vi "Table Stage GUI.vi"() -> ()   [LabVIEW 2014]
uses:
  Controls/Translation Stage Types.ctl
  Controls/Queue Manager Actions.ctl
  Controls/MessagePacket.ctl
  Controls/QueueNames.ctl
panel:
  in  "Control Panel":T1(tab)
  in  "Table Stage Motion Controls":enum32{"Table Stage Controls"}(tab)
  in  "X":dbl
  in  "Y":dbl
  in  "Z":dbl
  in  "dZ":dbl=0.1 min=0.1 step=0.1
  in  "dY":dbl=0.1 min=0.1 step=0.1
  in  "dX":dbl=0.1 min=0.1 step=0.1
  in  "+Y":bool
  in  "-X":bool
  in  "+X":bool
  in  "-Y":bool
  in  "+Z":bool
  in  "-Z":bool
  out "X Stage":bool
  out "Y Stage":bool
  out "Z Stage":bool
  in  "Mosaic Quick Nav.":bool[][](array[boolean])
  in  "X Stage 4":T2 caption="Device Type"
  in  "X Stage 3":T2 caption="Device Type"
  in  "Home 3":bool caption="Home"
  in  "Home 2":bool caption="Home"
  in  "Home":bool
  in  "Reconnect Z":bool caption="Reconnect"
  in  "Reconnect Y":bool caption="Reconnect"
  in  "Reconnect X":bool caption="Reconnect"
  in  "X Stage 2":T2 caption="Device Type"
  in  "Center Galvos":bool
  out "Error Out":errorcluster
  in  "Error In":errorcluster
  # "Stage Controls"
  # "XYZ Axis Control"
  # "Current Postion"
  # "X STAGE SETTINGS"
  # "Y STAGE SETTINGS"
  # "Z STAGE SETTINGS"
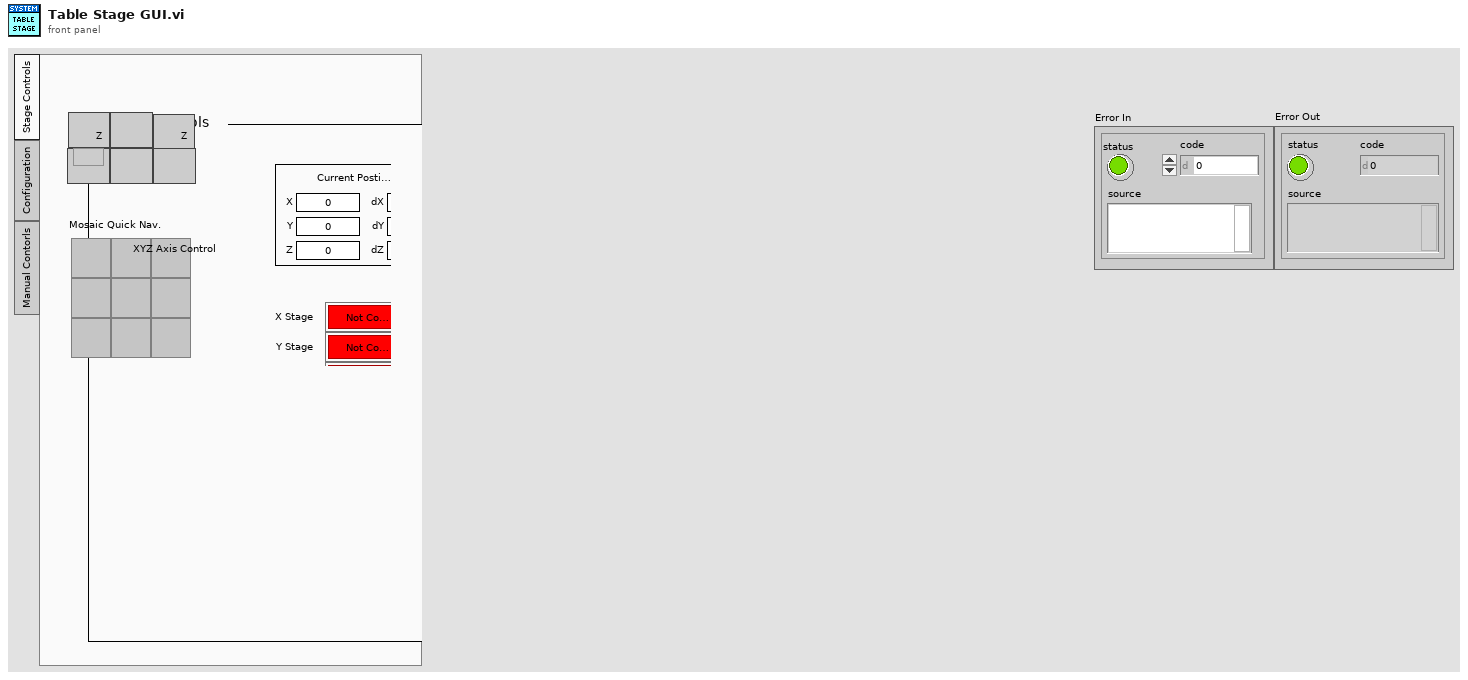
[diagram p1: front panel]
types:
  T1 = enum32{"Stage Controls", "Configuration", "Manual Contorls"}
  T2 = typedef "Translation Stage Types.ctl" = enum16{"None", "Thorlabs LTS", "Thorlabs MLJ"}
  T3 = typedef "MessagePacket.ctl" = cluster{"Message":string, "Parameter":variant}
  T4 = typedef "QueueNames.ctl" = enum16{"Main GUI", "Main Scan Processor", "Main Display", "Main Table Stage GUI", "Main Table Stage Proc."}
  T5 = typedef "Queue Manager Actions.ctl" = enum16{"Init", "Enqueue", "Enqueue All", "Preview Queue", "Dequeue", "Get Status", "Flush Queue", "Flush All Queues", "Release All Queues", "Release Queue"}
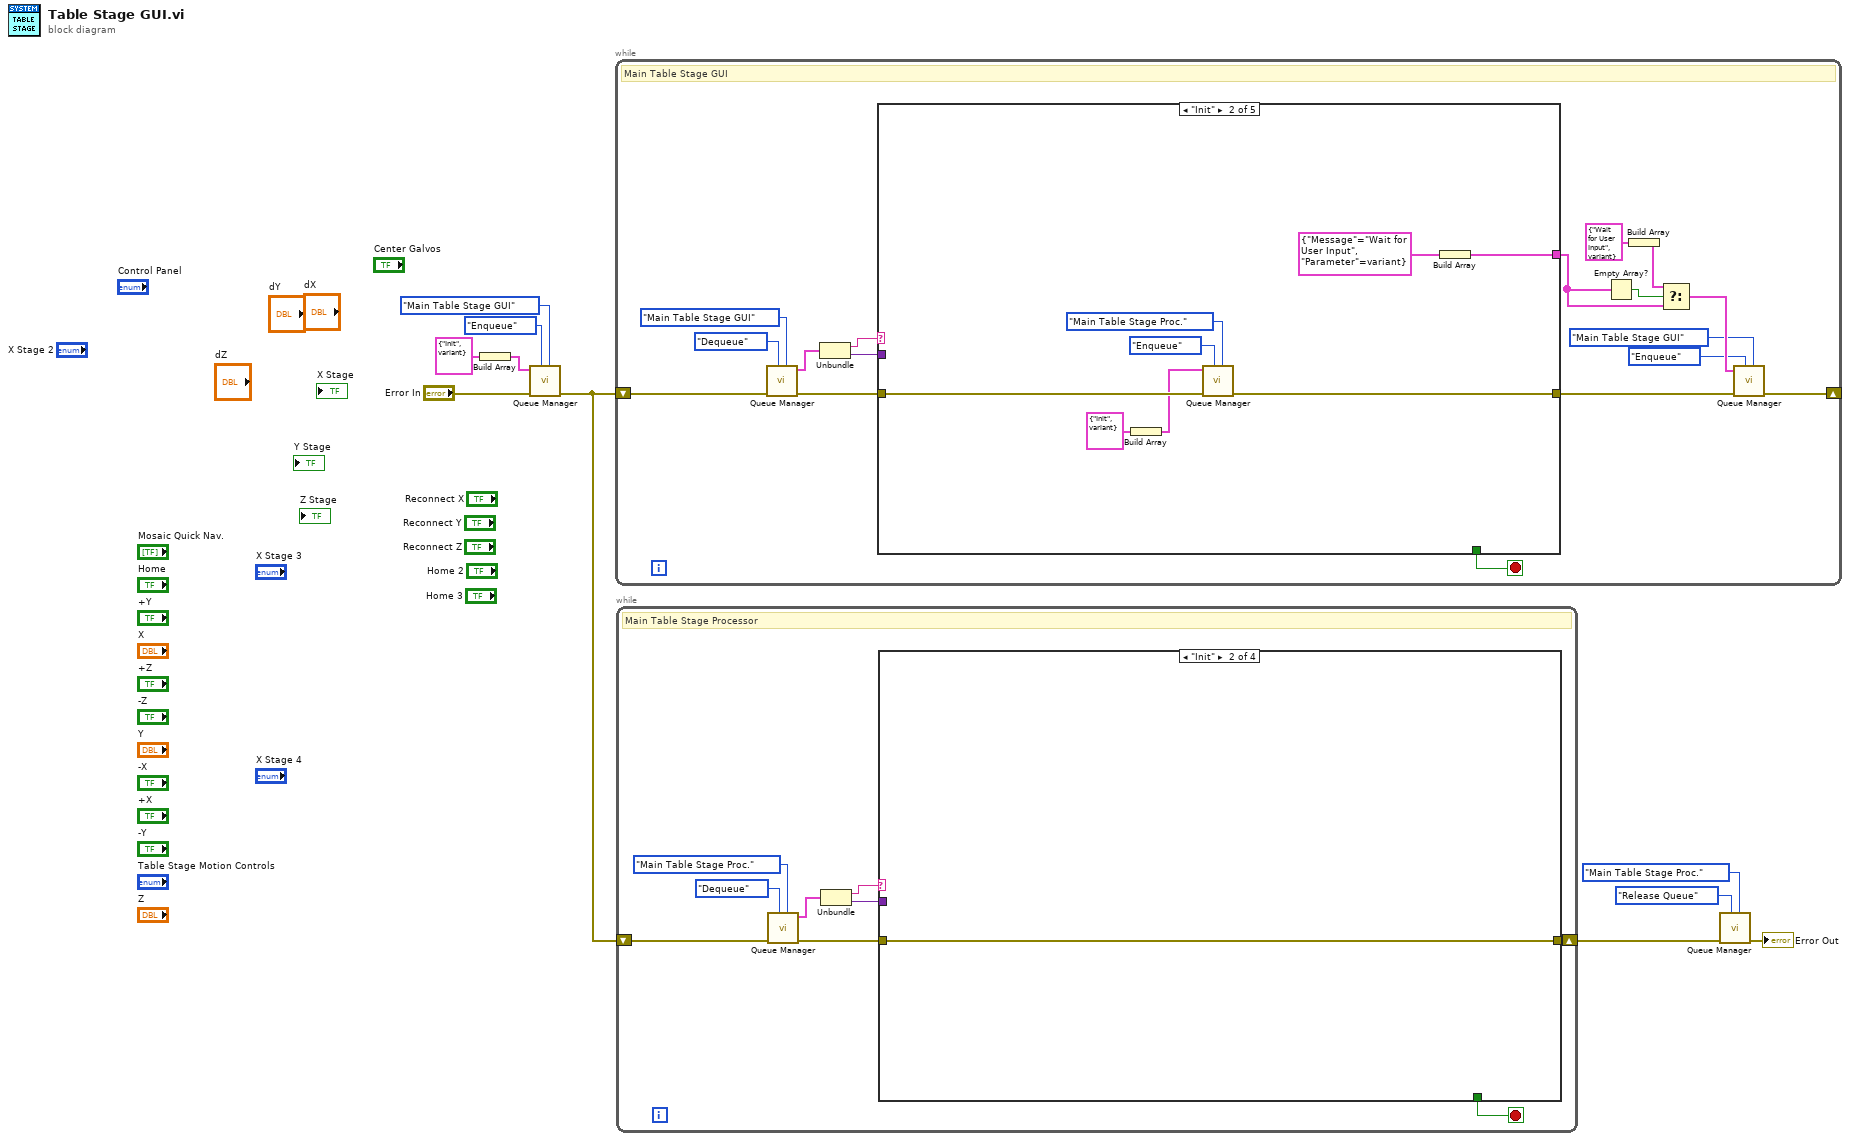
[diagram p0: block diagram]
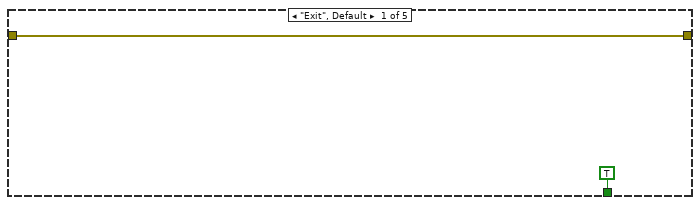
[diagram p2: hidden frame]
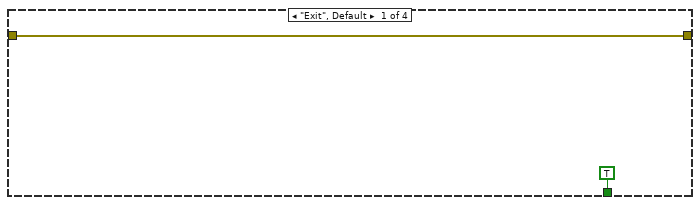
[diagram p6: hidden frame]
diagram:
  n1 = Build Array(T3 {"Message"="Init", "Parameter"=variant} ("Message Packet [In]")) -> (w1:T3[])
  n2 = call "Queue Manager.vi"("Queue Name"=QueueNames."Main Table Stage GUI", "Action"=Queue_Manager_Actions."Enqueue", "Error In"="Error In", "Message Packet Array"=w1) -> ("Error Out"=w3:errorcluster)  [unwired: 5 in, 2 out]
  n3 = while {
    shift-right: [w18] -> _
    shift-left: w3 -> [w25]
    stop <- w19 stop-if-true
    # "Main Table Stage GUI"
    n4 = call "Queue Manager.vi"("Queue Name"=QueueNames."Main Table Stage GUI", "Action"=Queue_Manager_Actions."Dequeue", "Error In"=w25) -> ("Error Out"=w24:errorcluster, "Message Packet [Out]"=w23:T3)  [unwired: 6 in, 1 out]
    n5 = Unbundle(w23) -> ("Message"=w22:string, "Parameter"=w21:variant)
    n6 = case shown="\"Init\"" w22 {
      tunnel: w24 -> [w28 w37 w38 w39 w40]
      tunnel: w21 -> [_ _ _ _ _]
      tunnel: [w28 w34 w38 w39 w40] -> w20
      tunnel: [TRUE _ _ _ _] -> w19
      tunnel: [_ w35 _ _ _] -> w11
      frame "Exit", Default {
      }
      frame "Init" {
        n7 = Build Array(T3 {"Message"="Init", "Parameter"=variant} ("Message Packet [In]")) -> (w30:T3[])
        n8 = call "Queue Manager.vi"("Queue Name"=QueueNames."Main Table Stage Proc.", "Action"=Queue_Manager_Actions."Enqueue", "Error In"=w37, "Message Packet Array"=w30) -> ("Error Out"=w34:errorcluster)  [unwired: 5 in, 2 out]
        n9 = Build Array(T3 {"Message"="Wait for User Input", "Parameter"=variant} ("Message Packet [In]")) -> (w35:T3[])
      }
      frame "Wait for User Input" {
      }
      frame "Init Hardware" {
      }
      frame "Idle" {
      }
    }
    n10 = Empty Array?(array=w11) -> (empty?=w17:bool)
    n11 = Build Array(T3 {"Message"="Wait for User Input", "Parameter"=variant} ("Message Packet [In]")) -> (w15:T3[])
    n12 = Select(t=w15, s=w17, f=w11) -> (s? t:f=w14:T3[])
    n13 = call "Queue Manager.vi"("Queue Name"=QueueNames."Main Table Stage GUI", "Action"=Queue_Manager_Actions."Enqueue", "Error In"=w20, "Message Packet Array"=w14) -> ("Error Out"=w18:errorcluster)  [unwired: 5 in, 2 out]
  }
  n14 = while {
    shift-right: [w42] -> w10
    shift-left: w3 -> [w47]
    stop <- w41 stop-if-true
    # "Main Table Stage Processor"
    n15 = call "Queue Manager.vi"("Queue Name"=QueueNames."Main Table Stage Proc.", "Action"=Queue_Manager_Actions."Dequeue", "Error In"=w47) -> ("Error Out"=w46:errorcluster, "Message Packet [Out]"=w45:T3)  [unwired: 6 in, 1 out]
    n16 = Unbundle(w45) -> ("Message"=w44:string, "Parameter"=w43:variant)
    n17 = case shown="\"Init\"" w44 {
      tunnel: w46 -> [w50 w52 w53 w54]
      tunnel: w43 -> [_ _ _ _]
      tunnel: [w50 w52 w53 w54] -> w42
      tunnel: [TRUE _ _ _] -> w41
      frame "Exit", Default {
      }
      frame "Init" {
      }
      frame "Init Hardware" {
      }
      frame "Idle" {
      }
    }
  }
  n18 = call "Queue Manager.vi"("Queue Name"=QueueNames."Main Table Stage Proc.", "Action"=Queue_Manager_Actions."Release Queue", "Error In"=w10) -> ("Error Out"=→"Error Out":errorcluster)  [unwired: 6 in, 2 out]
